vi "表格显示.vi"() -> ()   [LabVIEW 2013]
uses:
  <vilib>/Utility/config.llb/Config Data RefNum.ctl
  <vilib>/Utility/config.llb/NI_LVConfig.lvlib
panel:
  in  "油动机实验报告":T1
  in  "stop":bool
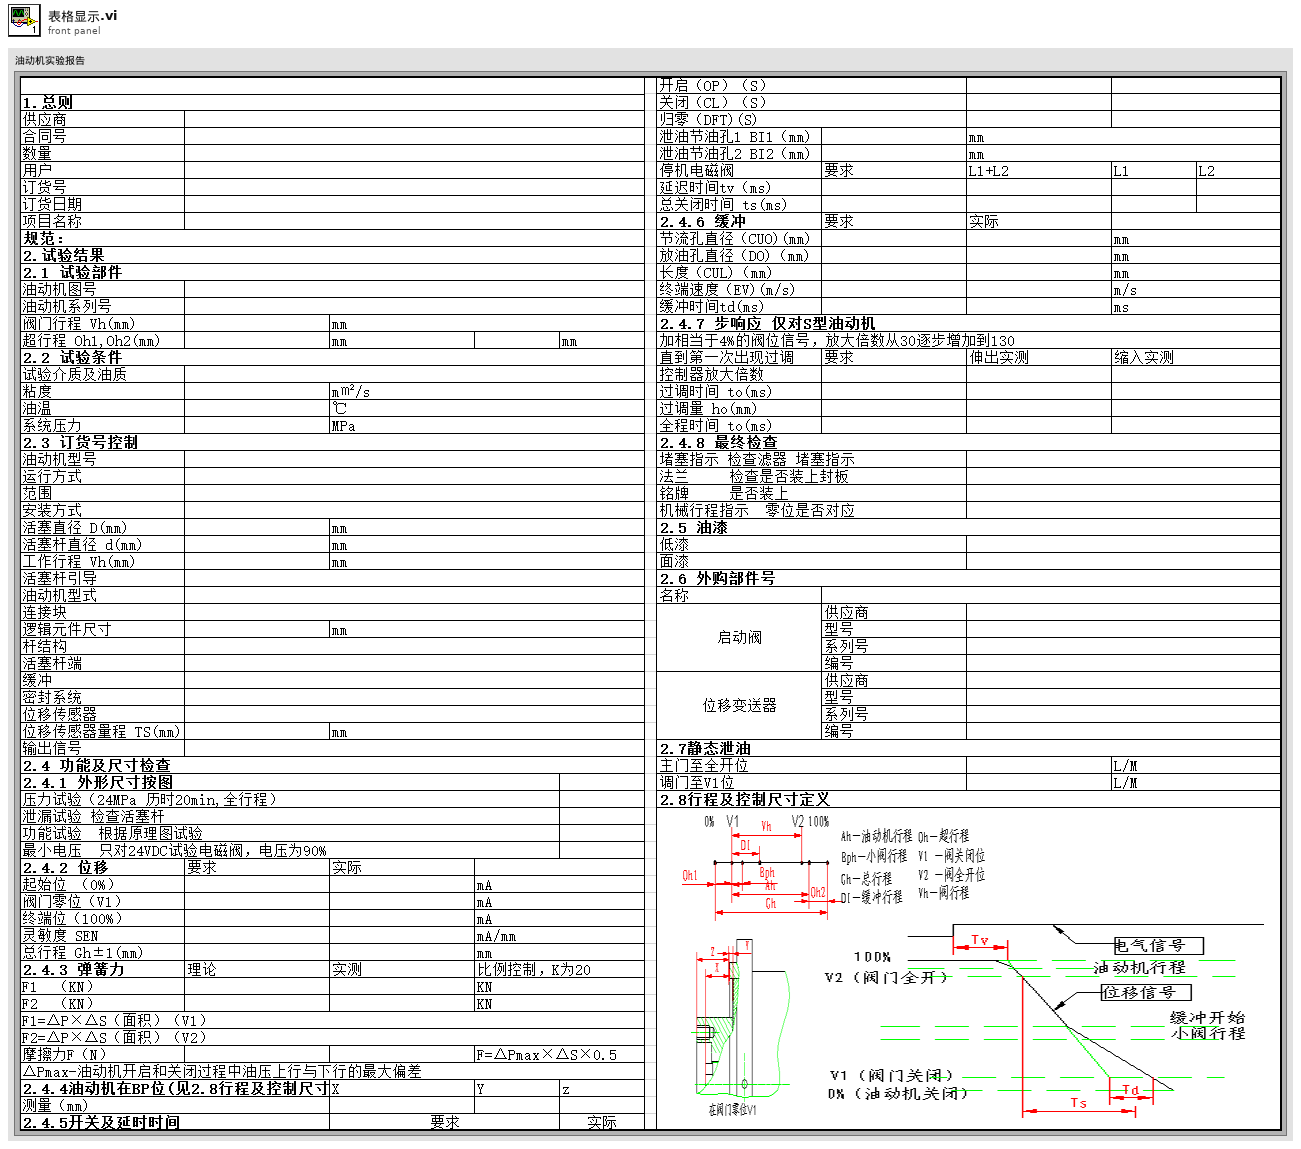
[diagram p1: front panel]
types:
  T1 = cluster{"供应商1":string, "合同号1":string, "数量1":string, "用户1":string, "订货号1":string, "订货日期1":string, "油动机图号2.1":string, "油动机系列号2.1":string, "阀门行程Vh":string, "试验介质及油质2.2":string, "超行程Oh1":string, "超行程Oh2":string, "粘度2.2":string, "油温2.2":string, "系统压力2.2":string, "油动机型号2.3":string, "运行方式2.3":string, "范围2.3":string, "安装方式2.3":string, "活塞直径D":string, "活塞杆直径d":string, "工作行程Vh2.3":string, "活塞杆引导2.3":string, "油动机型式2.3":string, "连接块2.3":string, "逻辑元件尺寸2.3":string, "杆结构2.3":string, "活塞杆端2.3":string, "缓冲2.3":string, "密封系统2.3":string, "位移传感器2.3":string, "位移传感器量程TS":string, "输出信号":string, "外形尺寸_2.4.1":string, "泄漏试验与否_2.4.1":string, "功能试验与否_2.4.1":string, "最小电压试验与否_2.4.1":string, "压力试验与否_2.4.1":string, "要求起始位2.4.2":string, "实际起始位":string, "要求总行程Gh2.4.2":string, "理论摩擦力F2.4.3":string, "要求灵敏度2.4.2":string, "理论F12.4.3":string, "要求终端位2.4.2":string, "要求阀门零位2.4.2":string, "理论F22.4.3":string, "实际阀门零位V1":string, "实际终端位V2":string, "实际灵敏度SEN":string, "实际总行程Gh":string, "实测F1":string, "实测F2":string, "实测F":string, "油动机在BP位_测量_X":string, "油动机在BP位_测量_Y":string, "油动机BP位_测量Z":string, "要求开关延时_开启2.4.5":string, "实际OP":string, "要求开关延时_关闭2.4.5":string, "实际CL":string, "要求开关延时_归零2.4.5":string, "实际DFT":string, "泄油节油孔1_BI1_2.4.5":string, "泄油节油孔2_BI2_2.4.5":string, "要求延迟时间tv_2.4.5":string, "要求总关闭时间ts_2.4.5":string, "要求_终端速度_2.4.6":string, "要求_长度_2.4.6":string, "要求_放油孔直径_2.4.6":string, "要求_节流孔直径_2.4.6":string, "延迟时间L1L2":string, "延迟时间L1":string, "延迟时间L2":string, "总关闭时间L1L2":string, "总关闭时间L1":string, "总关闭时间L2":string, "实际_节流孔直径_2.4.6":string, "缓冲时间td":string, "实际终端速度":string, "实际_长度_2.4.6":string, "实际_放油孔直径_2.4.6":string, "要求_缓冲时间_2.4.6":string, "控制器放大倍数_2.4.7":string, "伸出实测_控制器放大倍数_2.4.7":string, "缩入实测_控制器放大倍数_2.4.7":string, "要求_全程时间_2.4.7":string, "要求_过调时间_2.4.7":string, "要求_过调量_2.4.7":string, "伸出实测_全程时间":string, "伸出实测_过调量":string, "伸出实测_过调时间":string, "缩入实测_全程时间":string, "缩入实测_过调量":string, "缩入实测_过调时间":string, "堵塞指示_2.4.8":string, "法兰_2.4.8 ":string, "铭牌_2.4.8 ":string, "机械行程指示_2.4.8 ":string, "低漆_2.5":string, "面漆_2.5":string, "名称_2.6":string, "启动阀_供应商_2.6":string, "启动阀_型号_2.6":string, "启动阀_系列号_2.6":string, "启动阀_编号_2.6":string, "位移变送器_供应商_2.6":string, "位移变送器_型号_2.6":string, "位移变送器_系列号_2.6":string, "位移变送器_编号_2.6":string, "主门至全开位_2.7":string, "调门至V1位_2.7":string, "项目名称1":string, "油动机试验报告名称":string}
  T2 = typedef "NI_LVConfig.lvlib/Config Data RefNum.ctl" = refnum<k1>
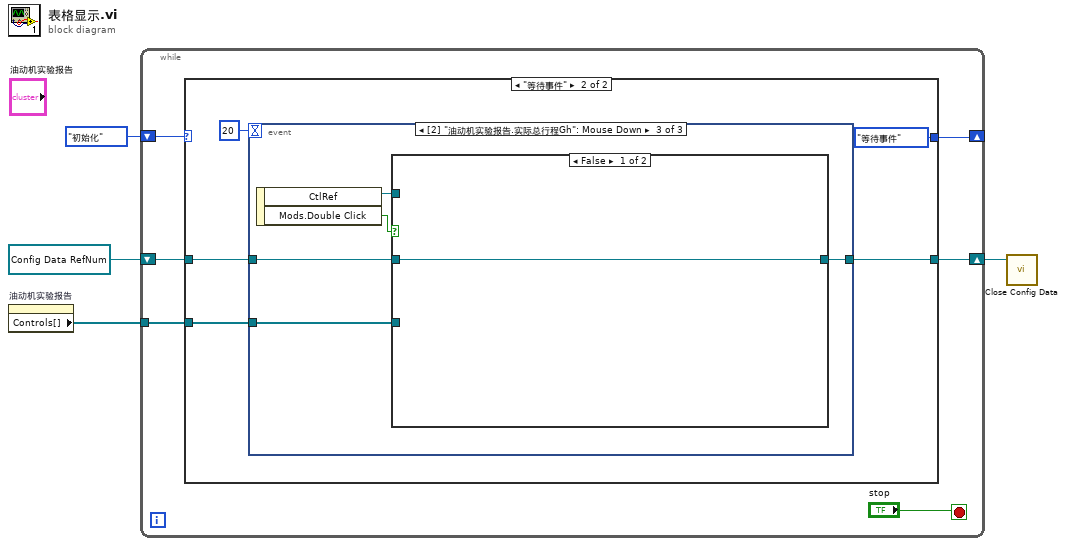
[diagram p0: block diagram]
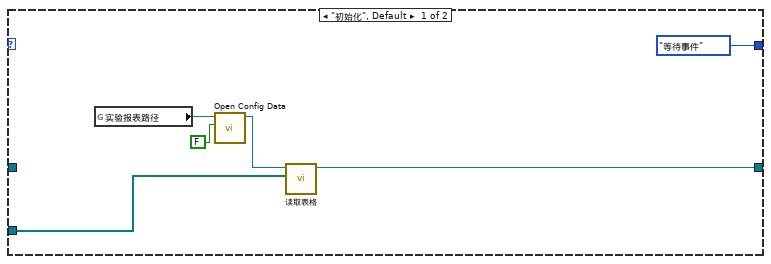
[diagram p2: hidden frame]
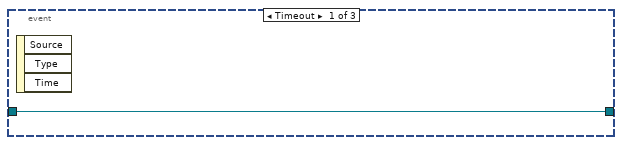
[diagram p3: hidden frame]
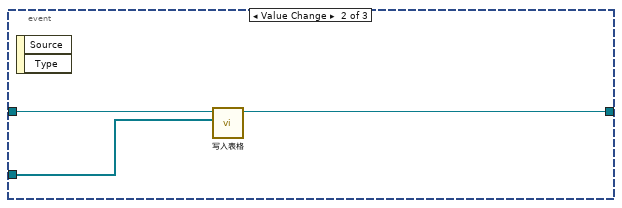
[diagram p4: hidden frame]
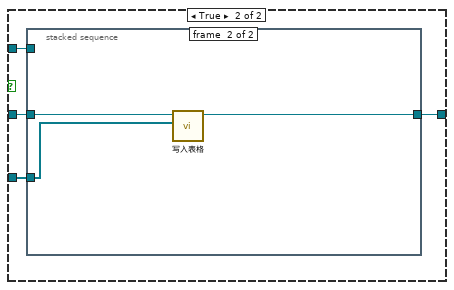
[diagram p5: hidden frame]
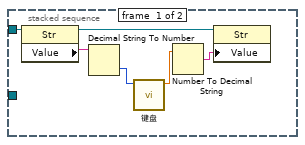
[diagram p6: hidden frame]
diagram:
  w3 = T2 refnum items=["config data"] ("引用句柄输入")
  n1 = property on="油动机实验报告" class="Clust (strict)"() -> ("Controls[]"=w1:refnum<vi>[])  [unwired: 2 in, 2 out]
  n2 = while {
    shift-right: [w8] -> _
    shift-left: enum16{"初始化", "等待事件"}."初始化" -> [w9]
    shift-right: [w7] -> w4
    shift-left: w3 -> [w5]
    tunnel: w1 -> [w6]
    stop <- "stop" stop-if-true
    n3 = case shown="\"等待事件\"" w9 {
      tunnel: [enum16{"初始化", "等待事件"}."等待事件" enum16{"初始化", "等待事件"}."等待事件"] -> w8
      tunnel: [w12 w17] -> w7
      tunnel: w6 -> [w11 w19]
      tunnel: w5 -> [_ w18]
      frame "初始化", Default {
        n4 = global read "实验报表路径.vi" "实验报表路径"() -> (w16:path)
        n5 = call <vilib>:"Open Config Data.vi"("create file if necessary (T)"=FALSE, "configuration file path"=w16) -> ("refnum"=w14:T2)  [unwired: 7 in, 2 out]
        n6 = call "读取表格.vi"("Controls[]"=w11, "引用句柄输入"=w14) -> ("引用句柄输出"=w12:T2)  [unwired: 8 in, 1 out]
      }
      frame "等待事件" {
        n7 = event shown="[2] \"油动机实验报告.实际总行程Gh\": Mouse Down" {
          selector: _ -> [_ _ _]
          dyn-events: _ -> [_ _ _]
          timeout: 20 -> [_ _ _]
          tunnel: w19 -> [_ w25 w27]
          tunnel: w18 -> [w22 w24 w28]
          tunnel: [w22 w23 w26] -> w17
          event Timeout {
            n8 = event-data() -> ()  [unwired: 1 in, 3 out]
          }
          event "油动机实验报告.用户1": Value Change {
            n9 = event-data() -> ()  [unwired: 1 in, 2 out]
            n10 = call "写入表格.vi"("Controls[]"=w25, "引用句柄输入"=w24) -> ("引用句柄输出"=w23:T2)  [unwired: 8 in, 1 out]
          }
          event "油动机实验报告.实际总行程Gh": Mouse Down {
            n11 = event-data() -> ("CtlRef"=w30:refnum<vi>, "Mods.Double Click"=w29:bool)  [unwired: 1 in]
            n12 = case shown="False" w29 {
              tunnel: w30 -> [_ w35]
              tunnel: w28 -> [w31 w34]
              tunnel: w27 -> [_ w33]
              tunnel: [w31 w32] -> w26
              frame False {
              }
              frame True {
                n13 = stacked-sequence {
                  tunnel: w35 -> [w41 _]
                  tunnel: w34 -> [_ w44]
                  tunnel: w33 -> [_ w43]
                  tunnel: [_ w42] -> w32
                  frame #0 {
                    n14 = property class="Str"(reference=w41) -> (reference out=w40:refnum<vi>, "Value"=w39:string)  [unwired: 1 in, 1 out]
                    n15 = Decimal String To Number(string=w39) -> (number=w38:i32)  [unwired: 2 in, 1 out]
                    n16 = call "键盘.vi"("原值"=w38) -> ("x+y"=w36:dbl)  [unwired: 10 in]
                    n17 = Number To Decimal String(number=w36) -> (decimal integer string=w37:string)  [unwired: 1 in]
                    n18 = property class="Str"(reference=w40, "Value"=w37) -> ()  [unwired: 1 in, 2 out]
                  }
                  frame #1 {
                    n19 = call "写入表格.vi"("Controls[]"=w43, "引用句柄输入"=w44) -> ("引用句柄输出"=w42:T2)  [unwired: 8 in, 1 out]
                  }
                }
              }
            }
          }
        }
      }
    }
  }
  n20 = call <vilib>:"Close Config Data.vi"("refnum"=w4) -> ()  [unwired: 9 in, 2 out]
